vi "InitGalvo.vi"(8 "error in":errorcluster, 10 "Output Array":dbl[](array[numeric])=[0.0], 11 "task/channels in":refnum<k21>) -> (0 "error out":errorcluster, 3 "task out":refnum<k21>)   [LabVIEW 2017]
doc: "This example demonstrates how to generate a user-defined voltage using the analog output of a DAQ device."
uses:
  <vilib>/DAQmx/write.llb/DAQmx Write (Analog 1D DBL NChan 1Samp).vi
  <vilib>/DAQmx/miscellaneous.llb/DAQmx Fill In Error Info.vi
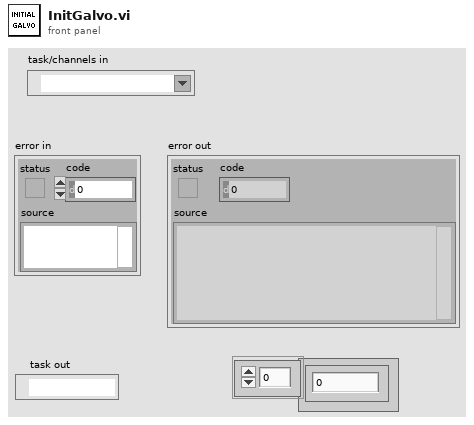
[diagram p1: front panel]
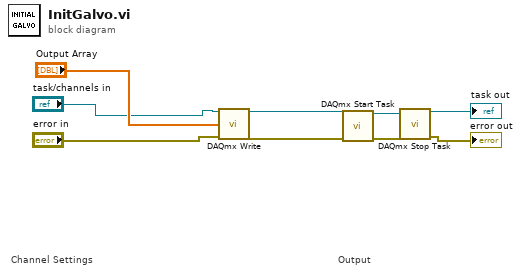
[diagram p0: block diagram]
diagram:
  # "Output"
  # "Channel Settings"
  n1 = call-poly <vilib>:"DAQmx Write.vi"("task/channels in"="task/channels in", "data"="Output Array", "error in"="error in") -> ("task out"=w5:refnum<k21>, "error out"=w6:errorcluster)  [unwired: 10 in, 1 out]
  n2 = call <vilib>:"DAQmx Start Task.vi"("task/channels in"=w5, "error in"=w6) -> ("task out"=w3:refnum<k21>, "error out"=w4:errorcluster)  [unwired: 12 in]
  n3 = call <vilib>:"DAQmx Stop Task.vi"("task/channels in"=w3, "error in"=w4) -> ("task out"=→"task out":refnum<k21>, "error out"=→"error out":errorcluster)  [unwired: 12 in]
